vi "Get LakeShore 340 PID.vi"(8 "error in (no error)":errorcluster, 10 "Output #":i32=1, 11 "VISA Resource Name":refnum<visa-resource-name>) -> (0 "error out":errorcluster, 1 "I":dbl, 2 "P":dbl, 3 "VISA Resource Name Out":refnum<visa-resource-name>, 4 "D":dbl)   [LabVIEW 2021]
uses:
  GPIB/VISA  Send Receive.vi
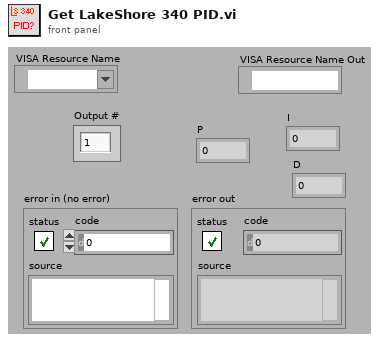
[diagram p1: front panel]
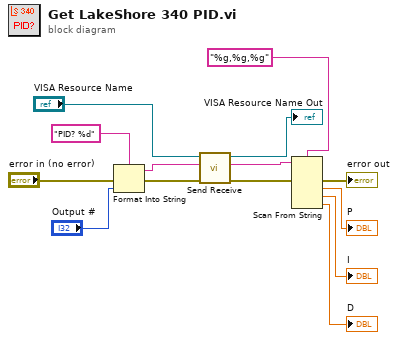
[diagram p0: block diagram]
diagram:
  n1 = Format Into String(format string="PID? %d" ("data string"), error in="error in (no error)", "Output #") -> (resulting string=w8:string, error out=w11:errorcluster)  [unwired: 1 in]
  n2 = call-poly "Send Receive.vi"("error in (no error)"=w11, "data string in"=w8, "VISA Resource Name"="VISA Resource Name") -> ("error out"=w5:errorcluster, "data string out"=w7:string, "VISA Resource Name Out"=→"VISA Resource Name Out":refnum<visa-resource-name>)  [unwired: 6 in]
  n3 = Scan From String(format string="%g,%g,%g", input string=w7, error in=w5) -> (error out=→"error out":errorcluster, output 1=→"P":dbl, output 2=→"I":dbl, output 3=→"D":dbl)  [unwired: 4 in, 2 out]
